vi "refresh C1 frequency.vi"(8 "error in (no error)":errorcluster, 11 "Waveform in":refnum<class "Waveform.lvclass">) -> (0 "error out":errorcluster, 3 "Waveform out":refnum<class "Waveform.lvclass">)   [LabVIEW 2012, in "Waveform.lvclass"]
uses:
  Waveform.lvclass
  Waveform.lvclass/Waveform.ctl
  <resource>/objmgr/daqmx.rc
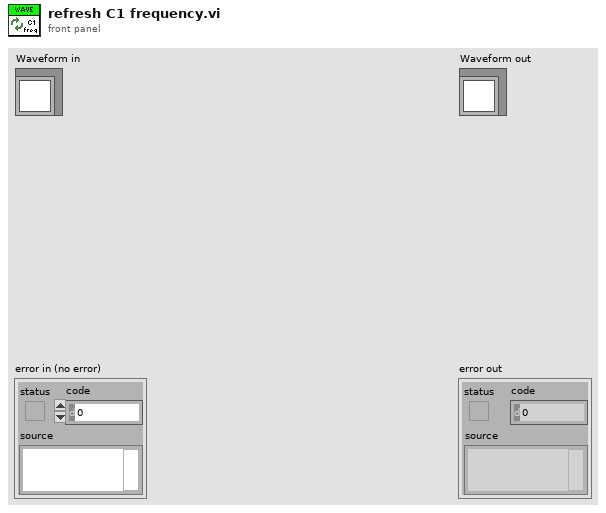
[diagram p1: front panel]
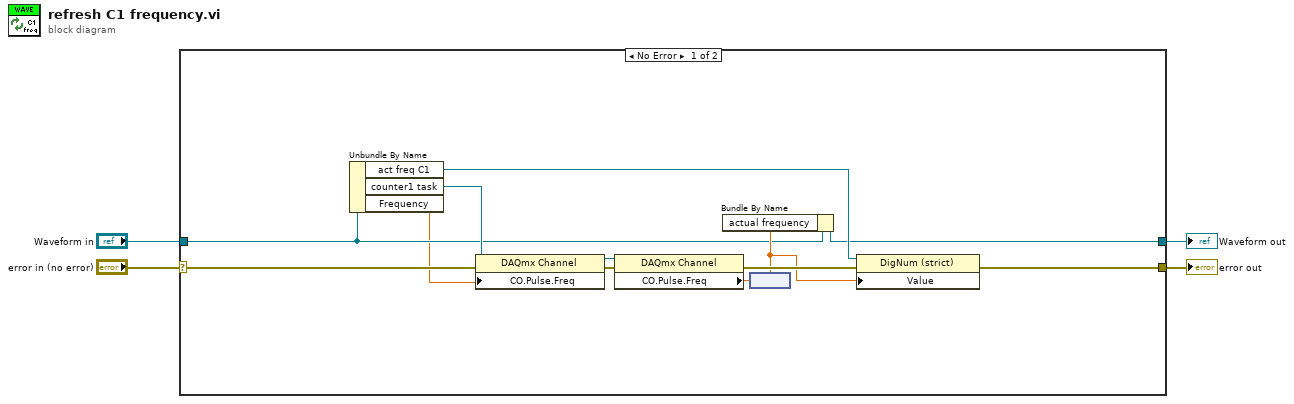
[diagram p0: block diagram]
diagram:
  n1 = case shown="No Error" "error in (no error)" {
    selector: "error in (no error)" -> [w7 w18]
    tunnel: [w6 w18] -> w3
    tunnel: [w8 w17] -> w1
    tunnel: "Waveform in" -> [w9 w17]
    frame No Error {
      n2 = Unbundle By Name(w9) -> ("act freq C1"=w11:refnum<vi>, "counter1 task"=w16:refnum<k21>, "Frequency"=w5:dbl)
      n3 = property class="DAQmx Channel"(reference=w16, error in=w7, "CO.Pulse.Freq"=w5) -> (reference out=w15:refnum<k21>, error out=w14:errorcluster)
      n4 = property class="DAQmx Channel"(reference=w15, error in=w14) -> (error out=w12:errorcluster, "CO.Pulse.Freq"=w13:dbl)  [unwired: 1 out]
      n5 = node(w13) -> (w10:dbl[unit])
      n6 = Bundle By Name(cluster=w9, "actual frequency"=w10) -> (w8:refnum<class "Waveform.lvclass">)
      n7 = property class="DigNum (strict)"(reference=w11, error in=w12, "Value"=w10) -> (error out=w6:errorcluster)  [unwired: 1 out]
    }
    frame Error {
    }
  }
  "error out" <- w3
  "Waveform out" <- w1
